vi "Test Simple Client.vi"() -> ()   [LabVIEW 2020]
uses:
  source/Client/Client/Client.lvclass
  source/Client/Subscription/Subscription.lvclass
  source/Client/Client/Put - I64.vi
  source/Client/Client/Put - U32.vi
  source/Client/Client/Put - I16.vi
  source/Client/Client/Put - U64.vi
  source/Client/Client/Put - U8.vi
  source/Client/Client/Put - I32.vi
  source/Client/Client/Put - U16.vi
  source/Client/Subscription/Next Value - U32.vi
  source/Client/Subscription/Next Value - I64.vi
  source/Client/Subscription/Next Value - U16.vi
  source/Client/Subscription/Next Value - U8.vi
  source/Client/Subscription/Next Value - I32.vi
  source/Client/Subscription/Next Value - I8.vi
  source/Client/Subscription/Next Value - U64.vi
  source/Client/Client/Put - I8.vi
  source/Client/Subscription/Next Value - I16.vi
panel:
  in  "U64":u64
  in  "U32":u32
  in  "U16":u16
  in  "U8":u8
  in  "I64":i64
  in  "I32":i32
  in  "I16":i16
  in  "I8":i8
  in  "stop":bool
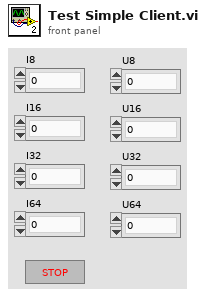
[diagram p1: front panel]
types:
  T1 = cluster{"PV name":string, "subscription":refnum<class "Subscription.lvclass">}
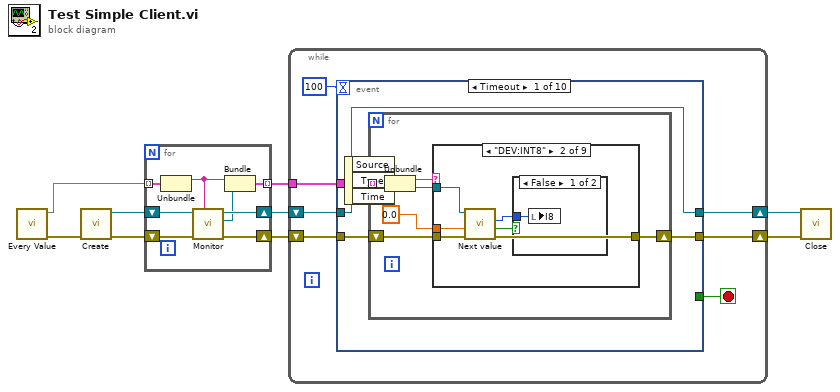
[diagram p0: block diagram]
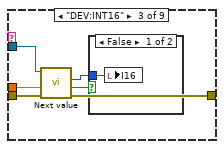
[diagram p4: hidden frame]
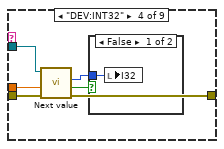
[diagram p6: hidden frame]
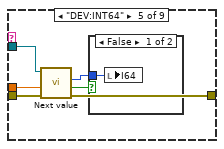
[diagram p8: hidden frame]
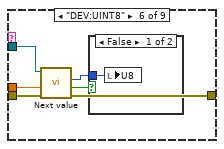
[diagram p10: hidden frame]
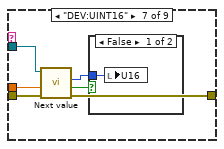
[diagram p12: hidden frame]
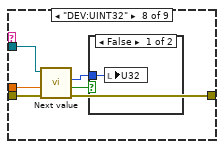
[diagram p14: hidden frame]
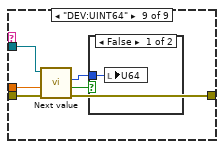
[diagram p16: hidden frame]
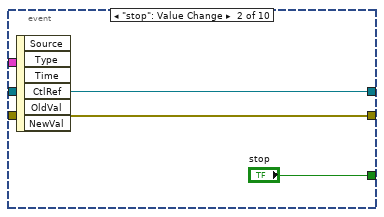
[diagram p18: hidden frame]
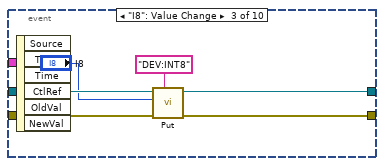
[diagram p19: hidden frame]
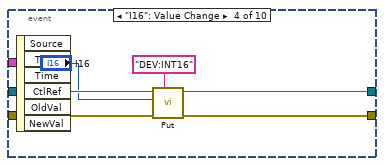
[diagram p20: hidden frame]
diagram:
  n1 = call "Every Value.vi"() -> ("error out"=w9:errorcluster, "values"=w6:map{string, refnum<class "NT Base.lvclass">})  [unwired: 10 in]
  n2 = call "Create.vi"("error in (no error)"=w9) -> ("error out"=w8:errorcluster, "Client out"=w7:refnum<class "Client.lvclass">)  [unwired: 9 in]
  n3 = for {
    tunnel: w6 -> [w15] mode=indexing
    shift-right: [w14] -> w5
    shift-left: w8 -> [w17]
    shift-right: [w13] -> w3
    shift-left: w7 -> [w16]
    tunnel: [w10] -> w4 mode=indexing
    n4 = Unbundle(w15) -> ("PV name"=w12:string)  [unwired: 1 out]
    n5 = call "Monitor.vi"("PV name"=w12, "error in"=w17, "Client in"=w16) -> ("error out"=w14:errorcluster, "subscription"=w11:refnum<class "Subscription.lvclass">, "Client out"=w13:refnum<class "Client.lvclass">)  [unwired: 6 in]
    n6 = Bundle("PV name"=w12, "subscription"=w11) -> (w10:T1)  [unwired: 1 in]
  }
  n7 = while {
    tunnel: w4 -> [w23]
    shift-right: [w22] -> w2
    shift-left: w5 -> [w24]
    shift-right: [w20] -> w1
    shift-left: w3 -> [w21]
    stop <- w19 stop-if-true
    n8 = event shown="[0] Timeout" {
      selector: _ -> [_ _ _ _ _ _ _ _ _ _]
      dyn-events: _ -> [_ _ _ _ _ _ _ _ _ _]
      timeout: 100 -> [_ _ _ _ _ _ _ _ _ _]
      tunnel: w24 -> [w28 w93 w100 w106 w112 w118 w124 w130 w136 w142]
      tunnel: w23 -> [w27 _ _ _ _ _ _ _ _ _]
      tunnel: [w26 w93 w99 w105 w111 w117 w123 w129 w135 w141] -> w22
      tunnel: w21 -> [w25 w92 w97 w103 w109 w115 w121 w127 w133 w139]
      tunnel: [w25 w92 w96 w102 w108 w114 w120 w126 w132 w138] -> w20
      tunnel: [_ "stop" _ _ _ _ _ _ _ _] -> w19
      event Timeout {
        n9 = event-data() -> ()  [unwired: 1 in, 3 out]
        n10 = for {
          tunnel: w27 -> [w34] mode=indexing
          shift-right: [w30] -> w26
          shift-left: w28 -> [w31]
          n11 = Unbundle(w34) -> ("PV name"=w33:string, "subscription"=w32:refnum<class "Subscription.lvclass">)
          n12 = case shown="\"DEV:INT8\"" w33 {
            tunnel: w32 -> [_ w41 w48 w55 w62 w69 w76 w83 w90]
            tunnel: w31 -> [w35 w40 w47 w54 w61 w68 w75 w82 w89]
            tunnel: [w35 w38 w45 w52 w59 w66 w73 w80 w87] -> w30
            tunnel: dbl[unit] 0.0 ("timeout") -> [_ w37 w44 w51 w58 w65 w72 w79 w86]
            frame Default {
            }
            frame "DEV:INT8" {
              n13 = call-poly "Next value.vi"("error in (no error)"=w40, "timeout"=w37, "Subscription in"=w41) -> ("error out"=w38:errorcluster, "timed out?"=w36:bool, "value"=w39:i8)  [unwired: 3 in, 3 out]
              n14 = case shown="False" w36 {
                tunnel: w39 -> [w42 _]
                frame False {
                  n15 = local write "I8"(w42) -> ()
                }
                frame True {
                }
              }
            }
            frame "DEV:INT16" {
              n16 = call-poly "Next value.vi"("error in (no error)"=w47, "timeout"=w44, "Subscription in"=w48) -> ("error out"=w45:errorcluster, "timed out?"=w43:bool, "value"=w46:i16)  [unwired: 3 in, 3 out]
              n17 = case shown="False" w43 {
                tunnel: w46 -> [w49 _]
                frame False {
                  n18 = local write "I16"(w49) -> ()
                }
                frame True {
                }
              }
            }
            frame "DEV:INT32" {
              n19 = call-poly "Next value.vi"("error in (no error)"=w54, "timeout"=w51, "Subscription in"=w55) -> ("error out"=w52:errorcluster, "timed out?"=w50:bool, "value"=w53:i32)  [unwired: 3 in, 3 out]
              n20 = case shown="False" w50 {
                tunnel: w53 -> [w56 _]
                frame False {
                  n21 = local write "I32"(w56) -> ()
                }
                frame True {
                }
              }
            }
            frame "DEV:INT64" {
              n22 = call-poly "Next value.vi"("error in (no error)"=w61, "timeout"=w58, "Subscription in"=w62) -> ("error out"=w59:errorcluster, "timed out?"=w57:bool, "value"=w60:i64)  [unwired: 3 in, 3 out]
              n23 = case shown="False" w57 {
                tunnel: w60 -> [w63 _]
                frame False {
                  n24 = local write "I64"(w63) -> ()
                }
                frame True {
                }
              }
            }
            frame "DEV:UINT8" {
              n25 = call-poly "Next value.vi"("error in (no error)"=w68, "timeout"=w65, "Subscription in"=w69) -> ("error out"=w66:errorcluster, "timed out?"=w64:bool, "value"=w67:u8)  [unwired: 3 in, 3 out]
              n26 = case shown="False" w64 {
                tunnel: w67 -> [w70 _]
                frame False {
                  n27 = local write "U8"(w70) -> ()
                }
                frame True {
                }
              }
            }
            frame "DEV:UINT16" {
              n28 = call-poly "Next value.vi"("error in (no error)"=w75, "timeout"=w72, "Subscription in"=w76) -> ("error out"=w73:errorcluster, "timed out?"=w71:bool, "value"=w74:u16)  [unwired: 3 in, 3 out]
              n29 = case shown="False" w71 {
                tunnel: w74 -> [w77 _]
                frame False {
                  n30 = local write "U16"(w77) -> ()
                }
                frame True {
                }
              }
            }
            frame "DEV:UINT32" {
              n31 = call-poly "Next value.vi"("error in (no error)"=w82, "timeout"=w79, "Subscription in"=w83) -> ("error out"=w80:errorcluster, "timed out?"=w78:bool, "value"=w81:u32)  [unwired: 3 in, 3 out]
              n32 = case shown="False" w78 {
                tunnel: w81 -> [w84 _]
                frame False {
                  n33 = local write "U32"(w84) -> ()
                }
                frame True {
                }
              }
            }
            frame "DEV:UINT64" {
              n34 = call-poly "Next value.vi"("error in (no error)"=w89, "timeout"=w86, "Subscription in"=w90) -> ("error out"=w87:errorcluster, "timed out?"=w85:bool, "value"=w88:u64)  [unwired: 3 in, 3 out]
              n35 = case shown="False" w85 {
                tunnel: w88 -> [w91 _]
                frame False {
                  n36 = local write "U64"(w91) -> ()
                }
                frame True {
                }
              }
            }
          }
        }
      }
      event "stop": Value Change {
        n37 = event-data() -> ()  [unwired: 1 in, 6 out]
      }
      event "I8": Value Change {
        n38 = event-data() -> ()  [unwired: 1 in, 6 out]
        n39 = call-poly "Put.vi"("PV name"="DEV:INT8", "error in (no error)"=w100, "value"="I8", "Client in"=w97) -> ("error out"=w99:errorcluster, "Client out"=w96:refnum<class "Client.lvclass">)  [unwired: 5 in, 1 out]
      }
      event "I16": Value Change {
        n40 = event-data() -> ()  [unwired: 1 in, 6 out]
        n41 = call-poly "Put.vi"("PV name"="DEV:INT16", "error in (no error)"=w106, "value"="I16", "Client in"=w103) -> ("error out"=w105:errorcluster, "Client out"=w102:refnum<class "Client.lvclass">)  [unwired: 5 in, 1 out]
      }
      event "I32": Value Change {
        n42 = event-data() -> ()  [unwired: 1 in, 6 out]
        n43 = call-poly "Put.vi"("PV name"="DEV:INT32", "error in (no error)"=w112, "value"="I32", "Client in"=w109) -> ("error out"=w111:errorcluster, "Client out"=w108:refnum<class "Client.lvclass">)  [unwired: 5 in, 1 out]
      }
      event "I64": Value Change {
        n44 = event-data() -> ()  [unwired: 1 in, 6 out]
        n45 = call-poly "Put.vi"("PV name"="DEV:INT64", "error in (no error)"=w118, "value"="I64", "Client in"=w115) -> ("error out"=w117:errorcluster, "Client out"=w114:refnum<class "Client.lvclass">)  [unwired: 5 in, 1 out]
      }
      event "U8": Value Change {
        n46 = event-data() -> ()  [unwired: 1 in, 6 out]
        n47 = call-poly "Put.vi"("PV name"="DEV:UINT8", "error in (no error)"=w124, "value"="U8", "Client in"=w121) -> ("error out"=w123:errorcluster, "Client out"=w120:refnum<class "Client.lvclass">)  [unwired: 5 in, 1 out]
      }
      event "U16": Value Change {
        n48 = event-data() -> ()  [unwired: 1 in, 6 out]
        n49 = call-poly "Put.vi"("PV name"="DEV:UINT16", "error in (no error)"=w130, "value"="U16", "Client in"=w127) -> ("error out"=w129:errorcluster, "Client out"=w126:refnum<class "Client.lvclass">)  [unwired: 5 in, 1 out]
      }
      event "U32": Value Change {
        n50 = event-data() -> ()  [unwired: 1 in, 6 out]
        n51 = call-poly "Put.vi"("PV name"="DEV:UINT32", "error in (no error)"=w136, "value"="U32", "Client in"=w133) -> ("error out"=w135:errorcluster, "Client out"=w132:refnum<class "Client.lvclass">)  [unwired: 5 in, 1 out]
      }
      event "U64": Value Change {
        n52 = event-data() -> ()  [unwired: 1 in, 6 out]
        n53 = call-poly "Put.vi"("PV name"="DEV:UINT64", "error in (no error)"=w142, "value"="U64", "Client in"=w139) -> ("error out"=w141:errorcluster, "Client out"=w138:refnum<class "Client.lvclass">)  [unwired: 5 in, 1 out]
      }
    }
  }
  n54 = call "Close.vi"("error in (no error)"=w2, "Client in"=w1) -> ()  [unwired: 9 in, 1 out]
